vi "Calculate X Y Step Size.vi"(6 "Overlap Options":T3 {"Percent Overlap" max=50}, 7 "Scan Pattern":T1(ring), 8 "Error In":errorcluster, 10 "Y Axis":T2, 11 "X Axis":T2) -> (0 "Error Out":errorcluster, 1 "Array":cluster{"X":dbl, "Y":dbl}[](array[cluster]), 2 "Y Axis Out":T2, 3 "X Axis Out":T2)   [LabVIEW 2018]
panel:
  out "XY Graph":cluster{"X":dbl, "Y":dbl}[](graph)
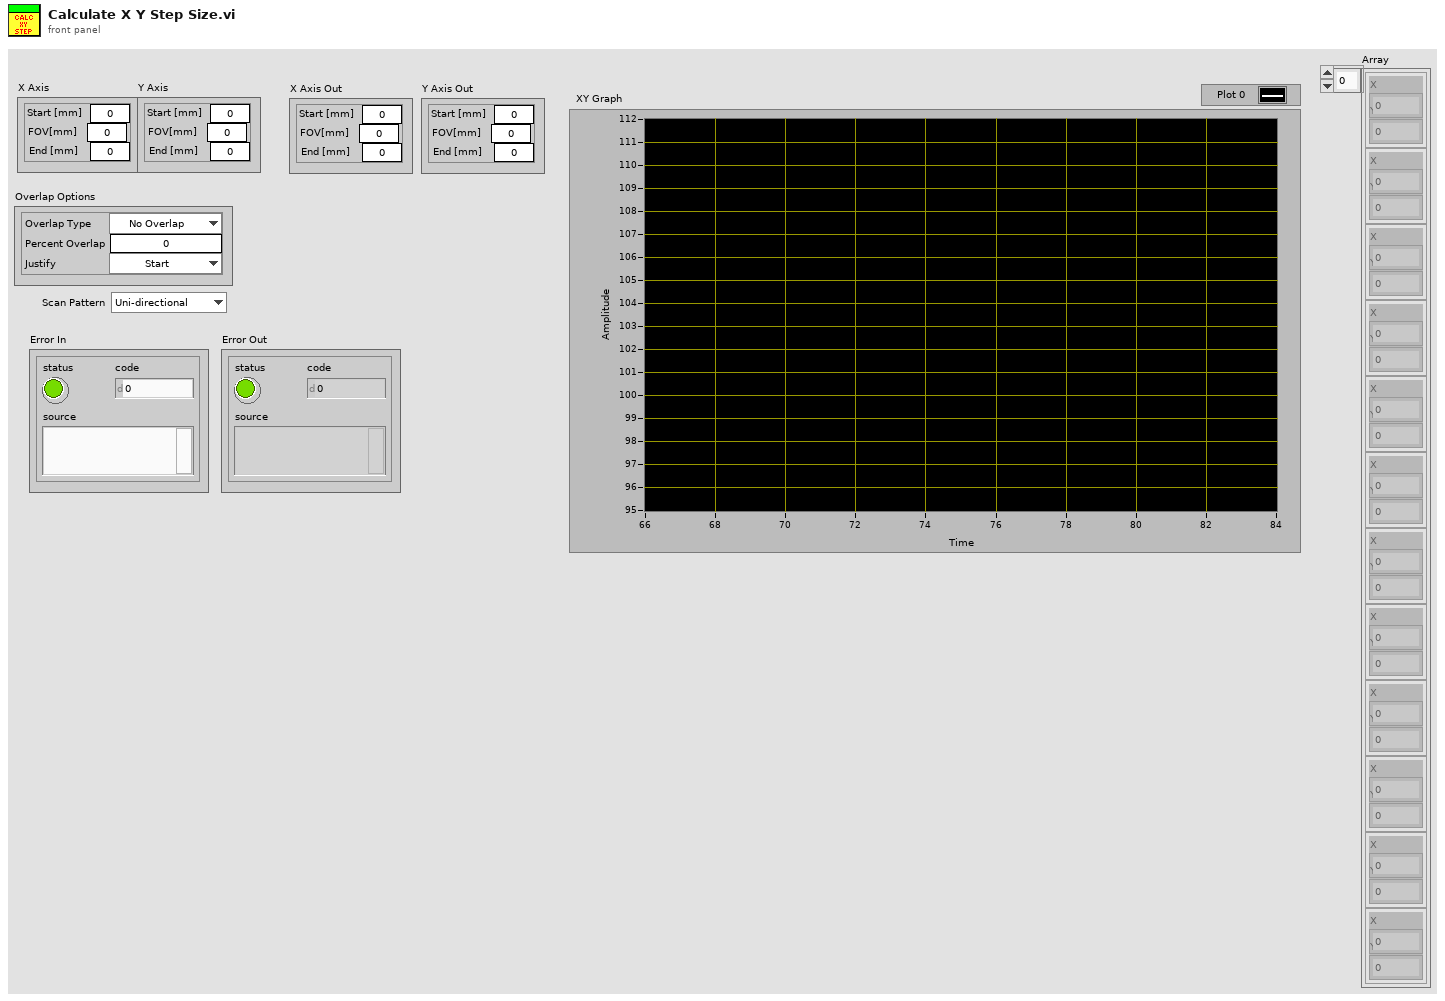
[diagram p1: front panel]
types:
  T1 = enum16{"Uni-directional", "Bi-Directional", "Spiral Out", "Spiral In"}
  T2 = cluster{"Start [mm]":dbl, "FOV[mm]":dbl, "End [mm]":dbl}
  T3 = cluster{"Overlap Type":enum16{"No Overlap", "X Only", "Y Only", "X and Y"}, "Percent Overlap":u8, "Justify":enum16{"Start", "Center", "End"}}
  T4 = enum16{"No Overlap", "X Only", "Y Only", "X and Y"}
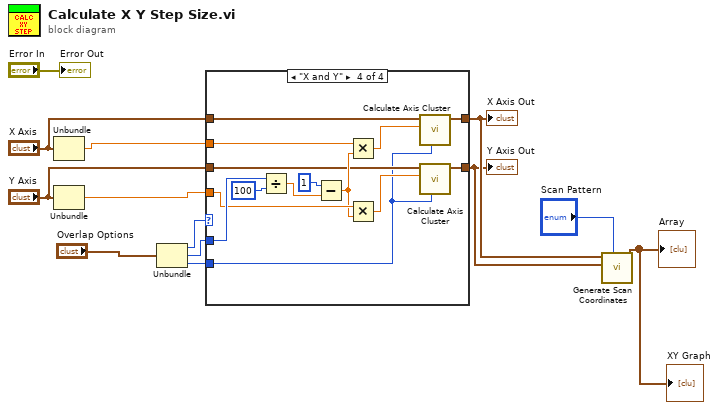
[diagram p0: block diagram]
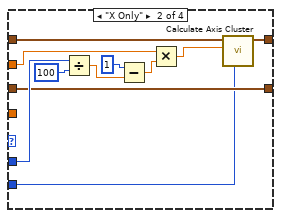
[diagram p3: hidden frame]
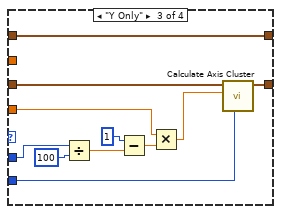
[diagram p4: hidden frame]
diagram:
  n1 = Unbundle("X Axis") -> ("FOV[mm]"=w2:dbl)  [unwired: 2 out]
  n2 = Unbundle("Y Axis") -> ("FOV[mm]"=w1:dbl)  [unwired: 2 out]
  n3 = Unbundle("Overlap Options") -> ("Overlap Type"=w12:T4, "Percent Overlap"=w11:u8, "Justify"=w7:enum16{"Start", "Center", "End"})
  n4 = case shown="\"X and Y\"" w12 {
    tunnel: w11 -> [_ w26 w37 w51]
    tunnel: w1 -> [_ _ w32 w47]
    tunnel: w2 -> [_ w22 _ w45]
    tunnel: "X Axis" -> [w15 w19 w31 w44]
    tunnel: "Y Axis" -> [w14 w20 w29 w43]
    tunnel: [w15 w17 w31 w40] -> w6
    tunnel: [w14 w20 w30 w39] -> w5
    tunnel: w7 -> [_ w16 w27 w38]
    frame "No Overlap", Default {
    }
    frame "X Only" {
      n5 = Divide(x=w26, y=u8 100) -> (x/y=w24:dbl)
      n6 = Subtract(x=u8 1 ("y"), y=w24) -> (x-y=w21:dbl)
      n7 = Multiply(x=w22, y=w21) -> (x*y=w18:dbl)
      n8 = call "Calculate Axis Cluster.vi"("Justify"=w16, "Step Size"=w18, "X Axis in"=w19) -> ("X Axis out"=w17:T2)  [unwired: 8 in]
    }
    frame "Y Only" {
      n9 = Divide(x=w37, y=u8 100) -> (x/y=w35:dbl)
      n10 = Subtract(x=u8 1 ("y"), y=w35) -> (x-y=w33:dbl)
      n11 = Multiply(x=w32, y=w33) -> (x*y=w28:dbl)
      n12 = call "Calculate Axis Cluster.vi"("Justify"=w27, "Step Size"=w28, "X Axis in"=w29) -> ("X Axis out"=w30:T2)  [unwired: 8 in]
    }
    frame "X and Y" {
      n13 = Divide(x=w51, y=u8 100) -> (x/y=w49:dbl)
      n14 = Subtract(x=u8 1 ("y"), y=w49) -> (x-y=w46:dbl)
      n15 = Multiply(x=w45, y=w46) -> (x*y=w42:dbl)
      n16 = Multiply(x=w47, y=w46) -> (x*y=w41:dbl)
      n17 = call "Calculate Axis Cluster.vi"("Justify"=w38, "Step Size"=w42, "X Axis in"=w44) -> ("X Axis out"=w40:T2)  [unwired: 8 in]
      n18 = call "Calculate Axis Cluster.vi"("Justify"=w38, "Step Size"=w41, "X Axis in"=w43) -> ("X Axis out"=w39:T2)  [unwired: 8 in]
    }
  }
  "X Axis Out" <- w6
  "Y Axis Out" <- w5
  n19 = call "Generate Scan Coordinates.vi"("Scan Pattern"="Scan Pattern", "Y Axis"=w5, "X Axis"=w6) -> ("Array"=→"XY Graph" →"Array":cluster{"X":dbl, "Y":dbl}[])  [unwired: 6 in, 2 out]
  "Error Out" <- "Error In"
